vi "诊断标定3 - 副本.vi"(8 "CAN端口":u16(ring), 9 "设备索引号":u16(ring), 10 "CAN卡类型":u32(ring)=21) -> ()   [LabVIEW 2013] (continued)
              tunnel: w2286 -> [w2289 w2294]
              tunnel: [w2289 w2293] -> w2285
              frame False {
              }
              frame True {
                n1897 = local write "布尔"(TRUE ("布尔")) -> ()
                n1898 = Enqueue Element(queue=w2296, element="读配置文件", error in (no error)=w2294) -> (queue out=w2295:refnum<queue>, error out=w2293:errorcluster)  [unwired: 2 out]
                n1899 = call <vilib>:"Set Busy.vi"() -> ()  [unwired: 4 in, 8 out]
              }
            }
          }
          event "保存主板参数": Value Change {
            n1900 = event-data() -> ("NewVal"=w2297:bool)  [unwired: 6 out]
            n1901 = case shown="真" w2297 {
              tunnel: w2301 -> [w2303 w2308]
              tunnel: [w2303 w2307] -> w2300
              tunnel: w2299 -> [w2302 w2306]
              tunnel: [w2302 w2305] -> w2298
              frame False {
              }
              frame True {
                n1902 = call <vilib>:"Set Busy.vi"() -> ()  [unwired: 4 in, 8 out]
                n1903 = Enqueue Element(queue=w2308, element="写配置文件", error in (no error)=w2306) -> (queue out=w2307:refnum<queue>, error out=w2305:errorcluster)  [unwired: 2 out]
              }
            }
          }
          event "继电器全开": Value Change {
            n1904 = event-data() -> ("NewVal"=w2309:bool)  [unwired: 6 out]
            n1905 = case shown="真" w2309 {
              tunnel: w2309 -> [_ w2312]
              frame False {
              }
              frame True {
                n1906 = stacked-sequence {
                  tunnel: w2312 -> [_ w2322 _]
                  frame #0 {
                    w2313 = FALSE ("清BUFF")
                    n1907 = local write "正级继电器"(w2313) -> ()
                    n1908 = local write "负级继电器"(w2313) -> ()
                    n1909 = local write "充电继电器"(w2313) -> ()
                    n1910 = local write "加热继电器"(w2313) -> ()
                    n1911 = local write "风机继电器"(w2313) -> ()
                    n1912 = local write "预充电继电器"(w2313) -> ()
                    n1913 = local write "继电器超时处理"(FALSE ("继电器超时处理")) -> ()
                    n1914 = local write "主从选择"(enum32{"主板", "从板"}."主板" ("主从选择")) -> ()
                    n1915 = local write "清BUFF"(FALSE ("清BUFF")) -> ()
                  }
                  frame #1 {
                    n1916 = case shown="真" w2322 {
                      selector: w2322 -> [_ w2337]
                      frame False {
                      }
                      frame True {
                        w2333 = 256.0 ("y")
                        w2324 = u32 1 ("命令序号")
                        w2323 = u8 192 ("命令")
                        n1917 = local read "动作保持时间"() -> (w2334:dbl)
                        n1918 = Quotient & Remainder(x=w2334, y=w2333) -> (x-y*floor(x/y)=w2326:dbl, floor(x/y)=w2330:dbl)
                        n1919 = Quotient & Remainder(x=w2330, y=w2333) -> (x-y*floor(x/y)=w2327:dbl, floor(x/y)=w2331:dbl)
                        n1920 = Quotient & Remainder(x=w2331, y=w2333) -> (x-y*floor(x/y)=w2328:dbl, floor(x/y)=w2332:dbl)
                        n1921 = local read "设备索引号"() -> (w2341:u16)
                        n1922 = local read "CAN卡类型"() -> (w2342:u32)
                        n1923 = local read "CAN端口"() -> (w2340:u16)
                        n1924 = Boolean To (0,1)(Boolean=w2337) -> (0, 1=w2335:i16)
                        n1925 = Quotient & Remainder(x=w2332, y=w2333) -> (x-y*floor(x/y)=w2329:dbl)  [unwired: 1 out]
                        n1926 = Build Array(i16 170 ("元素"), w2335, w2329, w2328, w2327, w2326, 0.0 ("元素")) -> (w2338:dbl[])
                        n1927 = call "多帧发送机制(EV05).vi"("can卡类型"=w2342, "设备索引号"=w2341, "CAN端口"=w2340, "命令"=w2323, "板号"=u8 0, "命令序号"=w2324, "输入数据"=w2338) -> ()  [unwired: 1 in, 12 out]
                        n1928 = local write "命令序号"(w2324) -> ()
                        n1929 = local write "命令"(w2323) -> ()
                      }
                    }
                    n1930 = local write "控制1"(TRUE ("控制1")) -> ()
                    n1931 = local write "写?"(FALSE ("写?")) -> ()
                    n1932 = local write "消除"(TRUE ("消除")) -> ()
                    n1933 = global write "EV05全局变量1.vi" "流控帧 2"(TRUE ("流控帧 2")) -> ()
                    n1934 = global write "EV05全局变量1.vi" "流控帧"(FALSE ("流控帧")) -> ()
                  }
                  frame #2 {
                    n1935 = flat-sequence {
                      tunnel: [w2344] -> w2343
                      tunnel: w2343 -> [w2351]
                      frame #0 {
                        n1936 = while {
                          tunnel: [w2345] -> w2344
                          i -> [w2349]
                          stop <- w2346 stop-if-true
                          n1937 = local read "继电器超时处理"() -> (w2345:bool)
                          n1938 = Greater Or Equal?(x=w2349, y=20) -> (x >= y?=w2347:bool)
                          n1939 = Wait Until Next ms Multiple(millisecond multiple=u32 100 ("毫秒倍数")) -> ()  [unwired: 1 out]
                          n1940 = Or(x=w2345, y=w2347) -> (x .or. y?=w2346:bool)
                        }
                      }
                      frame #1 {
                        n1941 = case shown="真" w2351 {
                          frame False {
                            n1942 = One Button Dialog(message="继电器处理超时" ("消息"), button name ("OK")="是" ("按钮名称（“确定”）")) -> ()  [unwired: 1 out]
                          }
                          frame True {
                            w2354 = TRUE ("清BUFF")
                            n1943 = local write "正级继电器"(w2354) -> ()
                            n1944 = local write "负级继电器"(w2354) -> ()
                            n1945 = local write "充电继电器"(w2354) -> ()
                            n1946 = local write "加热继电器"(w2354) -> ()
                            n1947 = local write "风机继电器"(w2354) -> ()
                            n1948 = local write "预充电继电器"(w2354) -> ()
                          }
                        }
                      }
                    }
                  }
                }
              }
            }
          }
          event "继电器全关": Value Change {
            n1949 = event-data() -> ("NewVal"=w2355:bool)  [unwired: 6 out]
            n1950 = case shown="真" w2355 {
              tunnel: w2355 -> [_ w2358]
              frame False {
              }
              frame True {
                n1951 = stacked-sequence {
                  tunnel: w2358 -> [_ w2368 _]
                  frame #0 {
                    w2359 = TRUE ("清BUFF")
                    n1952 = local write "正级继电器"(w2359) -> ()
                    n1953 = local write "负级继电器"(w2359) -> ()
                    n1954 = local write "充电继电器"(w2359) -> ()
                    n1955 = local write "加热继电器"(w2359) -> ()
                    n1956 = local write "风机继电器"(w2359) -> ()
                    n1957 = local write "预充电继电器"(w2359) -> ()
                    n1958 = local write "继电器超时处理"(FALSE ("继电器超时处理")) -> ()
                    n1959 = local write "主从选择"(enum32{"主板", "从板"}."主板" ("主从选择")) -> ()
                    n1960 = global write "EV05全局变量1.vi" "流控帧"(FALSE ("流控帧")) -> ()
                    n1961 = local write "清BUFF"(FALSE ("清BUFF")) -> ()
                  }
                  frame #1 {
                    n1962 = case shown="真" w2368 {
                      selector: w2368 -> [_ w2383]
                      frame False {
                      }
                      frame True {
                        w2379 = 256.0 ("y")
                        w2370 = u32 1 ("命令序号")
                        w2369 = u8 192 ("命令")
                        n1963 = local read "动作保持时间"() -> (w2380:dbl)
                        n1964 = Quotient & Remainder(x=w2380, y=w2379) -> (x-y*floor(x/y)=w2372:dbl, floor(x/y)=w2376:dbl)
                        n1965 = Quotient & Remainder(x=w2376, y=w2379) -> (x-y*floor(x/y)=w2373:dbl, floor(x/y)=w2377:dbl)
                        n1966 = Quotient & Remainder(x=w2377, y=w2379) -> (x-y*floor(x/y)=w2374:dbl, floor(x/y)=w2378:dbl)
                        n1967 = local read "设备索引号"() -> (w2387:u16)
                        n1968 = local read "CAN卡类型"() -> (w2388:u32)
                        n1969 = local read "CAN端口"() -> (w2386:u16)
                        n1970 = Boolean To (0,1)(Boolean=w2383) -> (0, 1=w2381:i16)
                        n1971 = Quotient & Remainder(x=w2378, y=w2379) -> (x-y*floor(x/y)=w2375:dbl)  [unwired: 1 out]
                        n1972 = Build Array(i16 85 ("元素"), w2381, w2375, w2374, w2373, w2372, 0.0 ("元素")) -> (w2384:dbl[])
                        n1973 = call "多帧发送机制(EV05).vi"("can卡类型"=w2388, "设备索引号"=w2387, "CAN端口"=w2386, "命令"=w2369, "板号"=u8 0, "命令序号"=w2370, "输入数据"=w2384) -> ()  [unwired: 1 in, 12 out]
                        n1974 = local write "命令序号"(w2370) -> ()
                        n1975 = local write "命令"(w2369) -> ()
                      }
                    }
                    n1976 = local write "控制1"(TRUE ("控制1")) -> ()
                    n1977 = local write "写?"(FALSE ("写?")) -> ()
                    n1978 = local write "消除"(TRUE ("消除")) -> ()
                    n1979 = global write "EV05全局变量1.vi" "流控帧 2"(TRUE ("流控帧 2")) -> ()
                  }
                  frame #2 {
                    n1980 = flat-sequence {
                      tunnel: [w2390] -> w2389
                      tunnel: w2389 -> [w2397]
                      frame #0 {
                        n1981 = while {
                          tunnel: [w2391] -> w2390
                          i -> [w2395]
                          stop <- w2392 stop-if-true
                          n1982 = local read "继电器超时处理"() -> (w2391:bool)
                          n1983 = Greater Or Equal?(x=w2395, y=20) -> (x >= y?=w2393:bool)
                          n1984 = Wait Until Next ms Multiple(millisecond multiple=u32 100 ("毫秒倍数")) -> ()  [unwired: 1 out]
                          n1985 = Or(x=w2391, y=w2393) -> (x .or. y?=w2392:bool)
                        }
                      }
                      frame #1 {
                        n1986 = case shown="真" w2397 {
                          frame False {
                            n1987 = One Button Dialog(message="继电器处理超时" ("消息"), button name ("OK")="是" ("按钮名称（“确定”）")) -> ()  [unwired: 1 out]
                          }
                          frame True {
                            w2400 = FALSE ("清BUFF")
                            n1988 = local write "正级继电器"(w2400) -> ()
                            n1989 = local write "负级继电器"(w2400) -> ()
                            n1990 = local write "充电继电器"(w2400) -> ()
                            n1991 = local write "加热继电器"(w2400) -> ()
                            n1992 = local write "风机继电器"(w2400) -> ()
                            n1993 = local write "预充电继电器"(w2400) -> ()
                          }
                        }
                      }
                    }
                  }
                }
              }
            }
          }
          event "控制按键全为开": Value Change {
            n1994 = event-data() -> ("NewVal"=w2401:bool)  [unwired: 6 out]
            n1995 = case shown="真" w2401 {
              frame False {
              }
              frame True {
                w2402 = TRUE ("正级继电器")
                n1996 = local write "加热继电器(从)"(w2402) -> ()
                n1997 = local write "风机继电器(从)"(w2402) -> ()
                n1998 = local write "DO1 2"(w2402) -> ()
                n1999 = local write "DO1"(w2402) -> ()
                n2000 = local write "DO2"(w2402) -> ()
                n2001 = local write "正级继电器"(w2402) -> ()
                n2002 = local write "负级继电器"(w2402) -> ()
                n2003 = local write "加热继电器"(w2402) -> ()
                n2004 = local write "预充电继电器"(w2402) -> ()
                n2005 = local write "充电继电器"(w2402) -> ()
                n2006 = local write "风机继电器"(w2402) -> ()
              }
            }
          }
          event "控制按键全为关": Value Change {
            n2007 = event-data() -> ("NewVal"=w2403:bool)  [unwired: 6 out]
            n2008 = case shown="真" w2403 {
              frame False {
              }
              frame True {
                w2404 = FALSE ("正级继电器")
                n2009 = local write "加热继电器(从)"(w2404) -> ()
                n2010 = local write "风机继电器(从)"(w2404) -> ()
                n2011 = local write "DO1 2"(w2404) -> ()
                n2012 = local write "DO1"(w2404) -> ()
                n2013 = local write "DO2"(w2404) -> ()
                n2014 = local write "正级继电器"(w2404) -> ()
                n2015 = local write "负级继电器"(w2404) -> ()
                n2016 = local write "加热继电器"(w2404) -> ()
                n2017 = local write "预充电继电器"(w2404) -> ()
                n2018 = local write "充电继电器"(w2404) -> ()
                n2019 = local write "风机继电器"(w2404) -> ()
              }
            }
          }
          event "正级继电器": Value Change {
            n2020 = event-data() -> ("NewVal"=w2405:bool)  [unwired: 6 out]
            n2021 = stacked-sequence {
              tunnel: w2405 -> [_ w2418 _]
              frame #0 {
                w2408 = FALSE ("清BUFF")
                n2022 = local write "继电器超时处理"(FALSE ("继电器超时处理")) -> ()
                n2023 = local write "主从选择"(enum32{"主板", "从板"}."主板" ("主从选择")) -> ()
                n2024 = local write "正级继电器 12"(w2408) -> ()
                n2025 = local write "清BUFF"(w2408) -> ()
              }
              frame #1 {
                n2026 = case shown="假" w2418 {
                  selector: w2418 -> [w2433 w2453]
                  tunnel: [w2432 w2452] -> w2417
                  tunnel: [w2420 w2440] -> w2412
                  frame False {
                    w2428 = 256.0 ("y")
                    w2420 = u32 1 ("命令序号")
                    w2432 = u8 192 ("命令")
                    n2027 = local read "动作保持时间"() -> (w2429:dbl)
                    n2028 = Quotient & Remainder(x=w2429, y=w2428) -> (x-y*floor(x/y)=w2421:dbl, floor(x/y)=w2425:dbl)
                    n2029 = Quotient & Remainder(x=w2425, y=w2428) -> (x-y*floor(x/y)=w2422:dbl, floor(x/y)=w2426:dbl)
                    n2030 = Quotient & Remainder(x=w2426, y=w2428) -> (x-y*floor(x/y)=w2423:dbl, floor(x/y)=w2427:dbl)
                    n2031 = local read "设备索引号"() -> (w2437:u16)
                    n2032 = local read "CAN卡类型"() -> (w2438:u32)
                    n2033 = local read "CAN端口"() -> (w2436:u16)
                    n2034 = Boolean To (0,1)(Boolean=w2433) -> (0, 1=w2430:i16)
                    n2035 = Quotient & Remainder(x=w2427, y=w2428) -> (x-y*floor(x/y)=w2424:dbl)  [unwired: 1 out]
                    n2036 = Build Array(i16 1 ("元素"), w2430, w2424, w2423, w2422, w2421, 0.0 ("元素")) -> (w2434:dbl[])
                    n2037 = call "多帧发送机制(EV05).vi"("can卡类型"=w2438, "设备索引号"=w2437, "CAN端口"=w2436, "命令"=w2432, "板号"=u8 0, "命令序号"=w2420, "输入数据"=w2434) -> ()  [unwired: 1 in, 12 out]
                  }
                  frame True {
                    w2448 = 256.0 ("y")
                    w2440 = u32 1 ("命令序号")
                    w2452 = u8 192 ("命令")
                    n2038 = local read "动作保持时间"() -> (w2449:dbl)
                    n2039 = Quotient & Remainder(x=w2449, y=w2448) -> (x-y*floor(x/y)=w2441:dbl, floor(x/y)=w2445:dbl)
                    n2040 = Quotient & Remainder(x=w2445, y=w2448) -> (x-y*floor(x/y)=w2442:dbl, floor(x/y)=w2446:dbl)
                    n2041 = Quotient & Remainder(x=w2446, y=w2448) -> (x-y*floor(x/y)=w2443:dbl, floor(x/y)=w2447:dbl)
                    n2042 = local read "设备索引号"() -> (w2457:u16)
                    n2043 = local read "CAN卡类型"() -> (w2458:u32)
                    n2044 = local read "CAN端口"() -> (w2456:u16)
                    n2045 = Boolean To (0,1)(Boolean=w2453) -> (0, 1=w2450:i16)
                    n2046 = Quotient & Remainder(x=w2447, y=w2448) -> (x-y*floor(x/y)=w2444:dbl)  [unwired: 1 out]
                    n2047 = Build Array(i16 1 ("元素"), w2450, w2444, w2443, w2442, w2441, 0.0 ("元素")) -> (w2454:dbl[])
                    n2048 = call "多帧发送机制(EV05).vi"("can卡类型"=w2458, "设备索引号"=w2457, "CAN端口"=w2456, "命令"=w2452, "板号"=u8 0, "命令序号"=w2440, "输入数据"=w2454) -> ()  [unwired: 1 in, 12 out]
                  }
                }
                n2049 = local write "命令序号"(w2412) -> ()
                n2050 = local write "命令"(w2417) -> ()
                n2051 = local write "控制1"(TRUE ("控制1")) -> ()
                n2052 = local write "写?"(FALSE ("写?")) -> ()
                n2053 = global write "EV05全局变量1.vi" "流控帧"(FALSE ("流控帧")) -> ()
                n2054 = local write "消除"(TRUE ("消除")) -> ()
                n2055 = global write "EV05全局变量1.vi" "流控帧 2"(TRUE ("流控帧 2")) -> ()
              }
              frame #2 {
                n2056 = flat-sequence {
                  tunnel: [w2460] -> w2459
                  tunnel: w2459 -> [w2467]
                  frame #0 {
                    n2057 = while {
                      tunnel: [w2461] -> w2460
                      i -> [w2465]
                      stop <- w2462 stop-if-true
                      n2058 = local read "继电器超时处理"() -> (w2461:bool)
                      n2059 = Greater Or Equal?(x=w2465, y=20) -> (x >= y?=w2463:bool)
                      n2060 = Wait Until Next ms Multiple(millisecond multiple=u32 100 ("毫秒倍数")) -> ()  [unwired: 1 out]
                      n2061 = Or(x=w2461, y=w2463) -> (x .or. y?=w2462:bool)
                    }
                  }
                  frame #1 {
                    n2062 = case shown="假" w2467 {
                      frame False {
                        n2063 = local read "正级继电器"() -> (w2469:bool)
                        n2064 = Not(x=w2469) -> (.not. x?=w2468:bool)
                        n2065 = local write "正级继电器"(w2468) -> ()
                        n2066 = One Button Dialog(message="继电器处理超时" ("消息"), button name ("OK")="是" ("按钮名称（“确定”）")) -> ()  [unwired: 1 out]
                      }
                      frame True {
                      }
                    }
                  }
                }
              }
            }
          }
          event "负级继电器": Value Change {
            n2067 = event-data() -> ("NewVal"=w2472:bool)  [unwired: 6 out]
            n2068 = stacked-sequence {
              tunnel: w2472 -> [_ w2485 _]
              frame #0 {
                w2475 = FALSE ("继电器超时处理")
                n2069 = local write "继电器超时处理"(w2475) -> ()
                n2070 = local write "正级继电器 2"(w2475) -> ()
                n2071 = local write "主从选择"(enum32{"主板", "从板"}."主板" ("主从选择")) -> ()
              }
              frame #1 {
                n2072 = case shown="假" w2485 {
                  selector: w2485 -> [w2499 w2519]
                  tunnel: [w2498 w2518] -> w2484
                  tunnel: [w2487 w2507] -> w2479
                  frame False {
                    w2495 = 256.0 ("y")
                    w2487 = u32 1 ("命令序号")
                    w2498 = u8 192 ("命令")
                    n2073 = local read "动作保持时间"() -> (w2496:dbl)
                    n2074 = Quotient & Remainder(x=w2496, y=w2495) -> (x-y*floor(x/y)=w2488:dbl, floor(x/y)=w2492:dbl)
                    n2075 = Quotient & Remainder(x=w2492, y=w2495) -> (x-y*floor(x/y)=w2489:dbl, floor(x/y)=w2493:dbl)
                    n2076 = Quotient & Remainder(x=w2493, y=w2495) -> (x-y*floor(x/y)=w2490:dbl, floor(x/y)=w2494:dbl)
                    n2077 = Quotient & Remainder(x=w2494, y=w2495) -> (x-y*floor(x/y)=w2491:dbl)  [unwired: 1 out]
                    n2078 = Boolean To (0,1)(Boolean=w2499) -> (0, 1=w2497:i16)
                    n2079 = local read "设备索引号"() -> (w2504:u16)
                    n2080 = local read "CAN卡类型"() -> (w2505:u32)
                    n2081 = local read "CAN端口"() -> (w2503:u16)
                    n2082 = Build Array(i16 2 ("元素"), w2497, w2491, w2490, w2489, w2488, 0.0 ("元素")) -> (w2501:dbl[])
                    n2083 = call "多帧发送机制(EV05).vi"("can卡类型"=w2505, "设备索引号"=w2504, "CAN端口"=w2503, "命令"=w2498, "板号"=u8 0, "命令序号"=w2487, "输入数据"=w2501) -> ()  [unwired: 1 in, 12 out]
                  }
                  frame True {
                    w2515 = 256.0 ("y")
                    w2507 = u32 1 ("命令序号")
                    w2518 = u8 192 ("命令")
                    n2084 = local read "动作保持时间"() -> (w2516:dbl)
                    n2085 = Quotient & Remainder(x=w2516, y=w2515) -> (x-y*floor(x/y)=w2508:dbl, floor(x/y)=w2512:dbl)
                    n2086 = Quotient & Remainder(x=w2512, y=w2515) -> (x-y*floor(x/y)=w2509:dbl, floor(x/y)=w2513:dbl)
                    n2087 = Quotient & Remainder(x=w2513, y=w2515) -> (x-y*floor(x/y)=w2510:dbl, floor(x/y)=w2514:dbl)
                    n2088 = Quotient & Remainder(x=w2514, y=w2515) -> (x-y*floor(x/y)=w2511:dbl)  [unwired: 1 out]
                    n2089 = Boolean To (0,1)(Boolean=w2519) -> (0, 1=w2517:i16)
                    n2090 = local read "设备索引号"() -> (w2524:u16)
                    n2091 = local read "CAN卡类型"() -> (w2525:u32)
                    n2092 = local read "CAN端口"() -> (w2523:u16)
                    n2093 = Build Array(i16 2 ("元素"), w2517, w2511, w2510, w2509, w2508, 0.0 ("元素")) -> (w2521:dbl[])
                    n2094 = call "多帧发送机制(EV05).vi"("can卡类型"=w2525, "设备索引号"=w2524, "CAN端口"=w2523, "命令"=w2518, "板号"=u8 0, "命令序号"=w2507, "输入数据"=w2521) -> ()  [unwired: 1 in, 12 out]
                  }
                }
                n2095 = local write "命令"(w2484) -> ()
                n2096 = local write "命令序号"(w2479) -> ()
                n2097 = local write "清BUFF"(FALSE ("清BUFF")) -> ()
                n2098 = global write "EV05全局变量1.vi" "流控帧"(FALSE ("流控帧")) -> ()
                n2099 = local write "控制1"(TRUE ("控制1")) -> ()
                n2100 = global write "EV05全局变量1.vi" "流控帧 2"(TRUE ("流控帧 2")) -> ()
                n2101 = local write "写?"(FALSE ("写?")) -> ()
                n2102 = local write "消除"(TRUE ("消除")) -> ()
              }
              frame #2 {
                n2103 = flat-sequence {
                  tunnel: [w2527] -> w2526
                  tunnel: w2526 -> [w2534]
                  frame #0 {
                    n2104 = while {
                      tunnel: [w2528] -> w2527
                      i -> [w2532]
                      stop <- w2529 stop-if-true
                      n2105 = local read "继电器超时处理"() -> (w2528:bool)
                      n2106 = Greater Or Equal?(x=w2532, y=20) -> (x >= y?=w2530:bool)
                      n2107 = Wait Until Next ms Multiple(millisecond multiple=u32 100 ("毫秒倍数")) -> ()  [unwired: 1 out]
                      n2108 = Or(x=w2528, y=w2530) -> (x .or. y?=w2529:bool)
                    }
                  }
                  frame #1 {
                    n2109 = case shown="假" w2534 {
                      frame False {
                        n2110 = local read "负级继电器"() -> (w2535:bool)
                        n2111 = Not(x=w2535) -> (.not. x?=w2536:bool)
                        n2112 = local write "负级继电器"(w2536) -> ()
                        n2113 = One Button Dialog(message="继电器处理超时" ("消息"), button name ("OK")="是" ("按钮名称（“确定”）")) -> ()  [unwired: 1 out]
                      }
                      frame True {
                      }
                    }
                  }
                }
              }
            }
          }
          event "预充电继电器": Value Change {
            n2114 = event-data() -> ("NewVal"=w2539:bool)  [unwired: 6 out]
            n2115 = stacked-sequence {
              tunnel: w2539 -> [_ w2552 _]
              frame #0 {
                w2543 = FALSE ("继电器超时处理")
                n2116 = local write "继电器超时处理"(w2543) -> ()
                n2117 = local write "正级继电器 3"(w2543) -> ()
                n2118 = global write "EV05全局变量1.vi" "流控帧"(FALSE ("流控帧")) -> ()
                n2119 = local write "主从选择"(enum32{"主板", "从板"}."主板" ("主从选择")) -> ()
              }
              frame #1 {
                n2120 = case shown="假" w2552 {
                  selector: w2552 -> [w2566 w2586]
                  tunnel: [w2565 w2585] -> w2551
                  tunnel: [w2554 w2574] -> w2546
                  frame False {
                    w2562 = 256.0 ("y")
                    w2554 = u32 1 ("命令序号")
                    w2565 = u8 192 ("命令")
                    n2121 = local read "动作保持时间"() -> (w2563:dbl)
                    n2122 = Quotient & Remainder(x=w2563, y=w2562) -> (x-y*floor(x/y)=w2555:dbl, floor(x/y)=w2559:dbl)
                    n2123 = Quotient & Remainder(x=w2559, y=w2562) -> (x-y*floor(x/y)=w2556:dbl, floor(x/y)=w2560:dbl)
                    n2124 = Quotient & Remainder(x=w2560, y=w2562) -> (x-y*floor(x/y)=w2557:dbl, floor(x/y)=w2561:dbl)
                    n2125 = Quotient & Remainder(x=w2561, y=w2562) -> (x-y*floor(x/y)=w2558:dbl)  [unwired: 1 out]
                    n2126 = Boolean To (0,1)(Boolean=w2566) -> (0, 1=w2564:i16)
                    n2127 = local read "设备索引号"() -> (w2571:u16)
                    n2128 = local read "CAN卡类型"() -> (w2572:u32)
                    n2129 = local read "CAN端口"() -> (w2570:u16)
                    n2130 = Build Array(i16 3 ("元素"), w2564, w2558, w2557, w2556, w2555, 0.0 ("元素")) -> (w2568:dbl[])
                    n2131 = call "多帧发送机制(EV05).vi"("can卡类型"=w2572, "设备索引号"=w2571, "CAN端口"=w2570, "命令"=w2565, "板号"=u8 0, "命令序号"=w2554, "输入数据"=w2568) -> ()  [unwired: 1 in, 12 out]
                  }
                  frame True {
                    w2582 = 256.0 ("y")
                    w2574 = u32 1 ("命令序号")
                    w2585 = u8 192 ("命令")
                    n2132 = local read "动作保持时间"() -> (w2583:dbl)
                    n2133 = Quotient & Remainder(x=w2583, y=w2582) -> (x-y*floor(x/y)=w2575:dbl, floor(x/y)=w2579:dbl)
                    n2134 = Quotient & Remainder(x=w2579, y=w2582) -> (x-y*floor(x/y)=w2576:dbl, floor(x/y)=w2580:dbl)
                    n2135 = Quotient & Remainder(x=w2580, y=w2582) -> (x-y*floor(x/y)=w2577:dbl, floor(x/y)=w2581:dbl)
                    n2136 = Quotient & Remainder(x=w2581, y=w2582) -> (x-y*floor(x/y)=w2578:dbl)  [unwired: 1 out]
                    n2137 = Boolean To (0,1)(Boolean=w2586) -> (0, 1=w2584:i16)
                    n2138 = local read "设备索引号"() -> (w2591:u16)
                    n2139 = local read "CAN卡类型"() -> (w2592:u32)
                    n2140 = local read "CAN端口"() -> (w2590:u16)
                    n2141 = Build Array(i16 3 ("元素"), w2584, w2578, w2577, w2576, w2575, 0.0 ("元素")) -> (w2588:dbl[])
                    n2142 = call "多帧发送机制(EV05).vi"("can卡类型"=w2592, "设备索引号"=w2591, "CAN端口"=w2590, "命令"=w2585, "板号"=u8 0, "命令序号"=w2574, "输入数据"=w2588) -> ()  [unwired: 1 in, 12 out]
                  }
                }
                n2143 = local write "命令序号"(w2546) -> ()
                n2144 = local write "清BUFF"(FALSE ("清BUFF")) -> ()
                n2145 = local write "控制1"(TRUE ("控制1")) -> ()
                n2146 = global write "EV05全局变量1.vi" "流控帧 2"(TRUE ("流控帧 2")) -> ()
                n2147 = local write "消除"(TRUE ("消除")) -> ()
                n2148 = local write "命令"(w2551) -> ()
                n2149 = local write "写?"(FALSE ("写?")) -> ()
              }
              frame #2 {
                n2150 = flat-sequence {
                  tunnel: [w2594] -> w2593
                  tunnel: w2593 -> [w2601]
                  frame #0 {
                    n2151 = while {
                      tunnel: [w2595] -> w2594
                      i -> [w2599]
                      stop <- w2596 stop-if-true
                      n2152 = local read "继电器超时处理"() -> (w2595:bool)
                      n2153 = Greater Or Equal?(x=w2599, y=20) -> (x >= y?=w2597:bool)
                      n2154 = Wait Until Next ms Multiple(millisecond multiple=u32 100 ("毫秒倍数")) -> ()  [unwired: 1 out]
                      n2155 = Or(x=w2595, y=w2597) -> (x .or. y?=w2596:bool)
                    }
                  }
                  frame #1 {
                    n2156 = case shown="假" w2601 {
                      frame False {
                        n2157 = local read "预充电继电器"() -> (w2602:bool)
                        n2158 = Not(x=w2602) -> (.not. x?=w2603:bool)
                        n2159 = local write "预充电继电器"(w2603) -> ()
                        n2160 = One Button Dialog(message="继电器处理超时" ("消息"), button name ("OK")="是" ("按钮名称（“确定”）")) -> ()  [unwired: 1 out]
                      }
                      frame True {
                      }
                    }
                  }
                }
              }
            }
          }
          event "加热继电器": Value Change {
            n2161 = event-data() -> ("NewVal"=w2606:bool)  [unwired: 6 out]
            n2162 = stacked-sequence {
              tunnel: w2606 -> [_ w2619 _]
              frame #0 {
                w2610 = FALSE ("继电器超时处理")
                n2163 = local write "继电器超时处理"(w2610) -> ()
                n2164 = local write "正级继电器 5"(w2610) -> ()
                n2165 = global write "EV05全局变量1.vi" "流控帧"(FALSE ("流控帧")) -> ()
                n2166 = local write "主从选择"(enum32{"主板", "从板"}."主板" ("主从选择")) -> ()
              }
              frame #1 {
                n2167 = case shown="假" w2619 {
                  selector: w2619 -> [w2633 w2653]
                  tunnel: [w2632 w2652] -> w2618
                  tunnel: [w2621 w2641] -> w2613
                  frame False {
                    w2629 = 256.0 ("y")
                    w2621 = u32 1 ("命令序号")
                    w2632 = u8 192 ("命令")
                    n2168 = local read "动作保持时间"() -> (w2630:dbl)
                    n2169 = Quotient & Remainder(x=w2630, y=w2629) -> (x-y*floor(x/y)=w2622:dbl, floor(x/y)=w2626:dbl)
                    n2170 = Quotient & Remainder(x=w2626, y=w2629) -> (x-y*floor(x/y)=w2623:dbl, floor(x/y)=w2627:dbl)
                    n2171 = Quotient & Remainder(x=w2627, y=w2629) -> (x-y*floor(x/y)=w2624:dbl, floor(x/y)=w2628:dbl)
                    n2172 = Quotient & Remainder(x=w2628, y=w2629) -> (x-y*floor(x/y)=w2625:dbl)  [unwired: 1 out]
                    n2173 = Boolean To (0,1)(Boolean=w2633) -> (0, 1=w2631:i16)
                    n2174 = local read "设备索引号"() -> (w2638:u16)
                    n2175 = local read "CAN卡类型"() -> (w2639:u32)
                    n2176 = local read "CAN端口"() -> (w2637:u16)
                    n2177 = Build Array(i16 4 ("元素"), w2631, w2625, w2624, w2623, w2622, 0.0 ("元素")) -> (w2635:dbl[])
                    n2178 = call "多帧发送机制(EV05).vi"("can卡类型"=w2639, "设备索引号"=w2638, "CAN端口"=w2637, "命令"=w2632, "板号"=u8 0, "命令序号"=w2621, "输入数据"=w2635) -> ()  [unwired: 1 in, 12 out]
                  }
                  frame True {
                    w2649 = 256.0 ("y")
                    w2641 = u32 1 ("命令序号")
                    w2652 = u8 192 ("命令")
                    n2179 = local read "动作保持时间"() -> (w2650:dbl)
                    n2180 = Quotient & Remainder(x=w2650, y=w2649) -> (x-y*floor(x/y)=w2642:dbl, floor(x/y)=w2646:dbl)
                    n2181 = Quotient & Remainder(x=w2646, y=w2649) -> (x-y*floor(x/y)=w2643:dbl, floor(x/y)=w2647:dbl)
                    n2182 = Quotient & Remainder(x=w2647, y=w2649) -> (x-y*floor(x/y)=w2644:dbl, floor(x/y)=w2648:dbl)
                    n2183 = Quotient & Remainder(x=w2648, y=w2649) -> (x-y*floor(x/y)=w2645:dbl)  [unwired: 1 out]
                    n2184 = Boolean To (0,1)(Boolean=w2653) -> (0, 1=w2651:i16)
                    n2185 = local read "设备索引号"() -> (w2658:u16)
                    n2186 = local read "CAN卡类型"() -> (w2659:u32)
                    n2187 = local read "CAN端口"() -> (w2657:u16)
                    n2188 = Build Array(i16 4 ("元素"), w2651, w2645, w2644, w2643, w2642, 0.0 ("元素")) -> (w2655:dbl[])
                    n2189 = call "多帧发送机制(EV05).vi"("can卡类型"=w2659, "设备索引号"=w2658, "CAN端口"=w2657, "命令"=w2652, "板号"=u8 0, "命令序号"=w2641, "输入数据"=w2655) -> ()  [unwired: 1 in, 12 out]
                  }
                }
                n2190 = local write "命令序号"(w2613) -> ()
                n2191 = local write "清BUFF"(FALSE ("清BUFF")) -> ()
                n2192 = local write "命令"(w2618) -> ()
                n2193 = local write "控制1"(TRUE ("控制1")) -> ()
                n2194 = local write "写?"(FALSE ("写?")) -> ()
                n2195 = global write "EV05全局变量1.vi" "流控帧 2"(TRUE ("流控帧 2")) -> ()
                n2196 = local write "消除"(TRUE ("消除")) -> ()
              }
              frame #2 {
                n2197 = flat-sequence {
                  tunnel: [w2661] -> w2660
                  tunnel: w2660 -> [w2668]
                  frame #0 {
                    n2198 = while {
                      tunnel: [w2662] -> w2661
                      i -> [w2666]
                      stop <- w2663 stop-if-true
                      n2199 = local read "继电器超时处理"() -> (w2662:bool)
                      n2200 = Greater Or Equal?(x=w2666, y=20) -> (x >= y?=w2664:bool)
                      n2201 = Wait Until Next ms Multiple(millisecond multiple=u32 100 ("毫秒倍数")) -> ()  [unwired: 1 out]
                      n2202 = Or(x=w2662, y=w2664) -> (x .or. y?=w2663:bool)
                    }
                  }
                  frame #1 {
                    n2203 = case shown="假" w2668 {
                      frame False {
                        n2204 = local read "加热继电器"() -> (w2669:bool)
                        n2205 = Not(x=w2669) -> (.not. x?=w2670:bool)
                        n2206 = local write "加热继电器"(w2670) -> ()
                        n2207 = One Button Dialog(message="继电器处理超时" ("消息"), button name ("OK")="是" ("按钮名称（“确定”）")) -> ()  [unwired: 1 out]
                      }
                      frame True {
                      }
                    }
                  }
                }
              }
            }
          }
          event "充电继电器": Value Change {
            n2208 = event-data() -> ("NewVal"=w2673:bool)  [unwired: 6 out]
            n2209 = stacked-sequence {
              tunnel: w2673 -> [_ w2686 _]
              frame #0 {
                w2677 = FALSE ("继电器超时处理")
                n2210 = local write "主从选择"(enum32{"主板", "从板"}."主板" ("主从选择")) -> ()
                n2211 = global write "EV05全局变量1.vi" "流控帧"(FALSE ("流控帧")) -> ()
                n2212 = local write "继电器超时处理"(w2677) -> ()
                n2213 = local write "正级继电器 4"(w2677) -> ()
              }
              frame #1 {
                n2214 = case shown="假" w2686 {
                  selector: w2686 -> [w2700 w2720]
                  tunnel: [w2699 w2719] -> w2685
                  tunnel: [w2688 w2708] -> w2680
                  frame False {
                    w2696 = 256.0 ("y")
                    w2688 = u32 1 ("命令序号")
                    w2699 = u8 192 ("命令")
                    n2215 = local read "动作保持时间"() -> (w2697:dbl)
                    n2216 = Quotient & Remainder(x=w2697, y=w2696) -> (x-y*floor(x/y)=w2689:dbl, floor(x/y)=w2693:dbl)
                    n2217 = Quotient & Remainder(x=w2693, y=w2696) -> (x-y*floor(x/y)=w2690:dbl, floor(x/y)=w2694:dbl)
                    n2218 = Quotient & Remainder(x=w2694, y=w2696) -> (x-y*floor(x/y)=w2691:dbl, floor(x/y)=w2695:dbl)
                    n2219 = Quotient & Remainder(x=w2695, y=w2696) -> (x-y*floor(x/y)=w2692:dbl)  [unwired: 1 out]
                    n2220 = Boolean To (0,1)(Boolean=w2700) -> (0, 1=w2698:i16)
                    n2221 = local read "设备索引号"() -> (w2705:u16)
                    n2222 = local read "CAN卡类型"() -> (w2706:u32)
                    n2223 = local read "CAN端口"() -> (w2704:u16)
                    n2224 = Build Array(i16 5 ("元素"), w2698, w2692, w2691, w2690, w2689, 0.0 ("元素")) -> (w2702:dbl[])
                    n2225 = call "多帧发送机制(EV05).vi"("can卡类型"=w2706, "设备索引号"=w2705, "CAN端口"=w2704, "命令"=w2699, "板号"=u8 0, "命令序号"=w2688, "输入数据"=w2702) -> ()  [unwired: 1 in, 12 out]
                  }
                  frame True {
                    w2716 = 256.0 ("y")
                    w2708 = u32 1 ("命令序号")
                    w2719 = u8 192 ("命令")
                    n2226 = local read "动作保持时间"() -> (w2717:dbl)
                    n2227 = Quotient & Remainder(x=w2717, y=w2716) -> (x-y*floor(x/y)=w2709:dbl, floor(x/y)=w2713:dbl)
                    n2228 = Quotient & Remainder(x=w2713, y=w2716) -> (x-y*floor(x/y)=w2710:dbl, floor(x/y)=w2714:dbl)
                    n2229 = Quotient & Remainder(x=w2714, y=w2716) -> (x-y*floor(x/y)=w2711:dbl, floor(x/y)=w2715:dbl)
                    n2230 = Quotient & Remainder(x=w2715, y=w2716) -> (x-y*floor(x/y)=w2712:dbl)  [unwired: 1 out]
                    n2231 = Boolean To (0,1)(Boolean=w2720) -> (0, 1=w2718:i16)
                    n2232 = local read "设备索引号"() -> (w2725:u16)
                    n2233 = local read "CAN卡类型"() -> (w2726:u32)
                    n2234 = local read "CAN端口"() -> (w2724:u16)
                    n2235 = Build Array(i16 5 ("元素"), w2718, w2712, w2711, w2710, w2709, 0.0 ("元素")) -> (w2722:dbl[])
                    n2236 = call "多帧发送机制(EV05).vi"("can卡类型"=w2726, "设备索引号"=w2725, "CAN端口"=w2724, "命令"=w2719, "板号"=u8 0, "命令序号"=w2708, "输入数据"=w2722) -> ()  [unwired: 1 in, 12 out]
                  }
                }
                n2237 = local write "命令序号"(w2680) -> ()
                n2238 = local write "命令"(w2685) -> ()
                n2239 = local write "清BUFF"(FALSE ("清BUFF")) -> ()
                n2240 = local write "控制1"(TRUE ("控制1")) -> ()
                n2241 = global write "EV05全局变量1.vi" "流控帧 2"(TRUE ("流控帧 2")) -> ()
                n2242 = local write "写?"(FALSE ("写?")) -> ()
                n2243 = local write "消除"(TRUE ("消除")) -> ()
              }
              frame #2 {
                n2244 = flat-sequence {
                  tunnel: [w2728] -> w2727
                  tunnel: w2727 -> [w2735]
                  frame #0 {
                    n2245 = while {
                      tunnel: [w2729] -> w2728
                      i -> [w2733]
                      stop <- w2730 stop-if-true
                      n2246 = local read "继电器超时处理"() -> (w2729:bool)
                      n2247 = Greater Or Equal?(x=w2733, y=20) -> (x >= y?=w2731:bool)
                      n2248 = Wait Until Next ms Multiple(millisecond multiple=u32 100 ("毫秒倍数")) -> ()  [unwired: 1 out]
                      n2249 = Or(x=w2729, y=w2731) -> (x .or. y?=w2730:bool)
                    }
                  }
                  frame #1 {
                    n2250 = case shown="假" w2735 {
                      frame False {
                        n2251 = local read "充电继电器"() -> (w2736:bool)
                        n2252 = Not(x=w2736) -> (.not. x?=w2737:bool)
                        n2253 = local write "充电继电器"(w2737) -> ()
                        n2254 = One Button Dialog(message="继电器处理超时" ("消息"), button name ("OK")="是" ("按钮名称（“确定”）")) -> ()  [unwired: 1 out]
                      }
                      frame True {
                      }
                    }
                  }
                }
              }
            }
          }
          event "风机继电器": Value Change {
            n2255 = event-data() -> ("NewVal"=w2740:bool)  [unwired: 6 out]
            n2256 = stacked-sequence {
              tunnel: w2740 -> [_ w2753 _]
              frame #0 {
                w2744 = FALSE ("继电器超时处理")
                n2257 = local write "继电器超时处理"(w2744) -> ()
                n2258 = local write "正级继电器 6"(w2744) -> ()
                n2259 = global write "EV05全局变量1.vi" "流控帧"(FALSE ("流控帧")) -> ()
                n2260 = local write "主从选择"(enum32{"主板", "从板"}."主板" ("主从选择")) -> ()
              }
              frame #1 {
                n2261 = case shown="真" w2753 {
                  selector: w2753 -> [w2767 w2787]
                  tunnel: [w2766 w2786] -> w2752
                  tunnel: [w2755 w2775] -> w2747
                  frame True {
                    w2763 = 256.0 ("y")
                    w2755 = u32 1 ("命令序号")
                    w2766 = u8 192 ("命令")
                    n2262 = local read "动作保持时间"() -> (w2764:dbl)
                    n2263 = Quotient & Remainder(x=w2764, y=w2763) -> (x-y*floor(x/y)=w2756:dbl, floor(x/y)=w2760:dbl)
                    n2264 = Quotient & Remainder(x=w2760, y=w2763) -> (x-y*floor(x/y)=w2757:dbl, floor(x/y)=w2761:dbl)
                    n2265 = Quotient & Remainder(x=w2761, y=w2763) -> (x-y*floor(x/y)=w2758:dbl, floor(x/y)=w2762:dbl)
                    n2266 = Boolean To (0,1)(Boolean=w2767) -> (0, 1=w2765:i16)
                    n2267 = local read "设备索引号"() -> (w2772:u16)
                    n2268 = local read "CAN卡类型"() -> (w2773:u32)
                    n2269 = Quotient & Remainder(x=w2762, y=w2763) -> (x-y*floor(x/y)=w2759:dbl)  [unwired: 1 out]
                    n2270 = local read "CAN端口"() -> (w2771:u16)
                    n2271 = Build Array(i16 6 ("元素"), w2765, w2759, w2758, w2757, w2756, 0.0 ("元素")) -> (w2769:dbl[])
                    n2272 = call "多帧发送机制(EV05).vi"("can卡类型"=w2773, "设备索引号"=w2772, "CAN端口"=w2771, "命令"=w2766, "板号"=u8 0, "命令序号"=w2755, "输入数据"=w2769) -> ()  [unwired: 1 in, 12 out]
                  }
                  frame False {
                    w2783 = 256.0 ("y")
                    w2775 = u32 1 ("命令序号")
                    w2786 = u8 192 ("命令")
                    n2273 = local read "动作保持时间"() -> (w2784:dbl)
                    n2274 = Quotient & Remainder(x=w2784, y=w2783) -> (x-y*floor(x/y)=w2776:dbl, floor(x/y)=w2780:dbl)
                    n2275 = Quotient & Remainder(x=w2780, y=w2783) -> (x-y*floor(x/y)=w2777:dbl, floor(x/y)=w2781:dbl)
                    n2276 = Quotient & Remainder(x=w2781, y=w2783) -> (x-y*floor(x/y)=w2778:dbl, floor(x/y)=w2782:dbl)
                    n2277 = Boolean To (0,1)(Boolean=w2787) -> (0, 1=w2785:i16)
                    n2278 = local read "设备索引号"() -> (w2792:u16)
                    n2279 = local read "CAN卡类型"() -> (w2793:u32)
                    n2280 = Quotient & Remainder(x=w2782, y=w2783) -> (x-y*floor(x/y)=w2779:dbl)  [unwired: 1 out]
                    n2281 = local read "CAN端口"() -> (w2791:u16)
                    n2282 = Build Array(i16 6 ("元素"), w2785, w2779, w2778, w2777, w2776, 0.0 ("元素")) -> (w2789:dbl[])
                    n2283 = call "多帧发送机制(EV05).vi"("can卡类型"=w2793, "设备索引号"=w2792, "CAN端口"=w2791, "命令"=w2786, "板号"=u8 0, "命令序号"=w2775, "输入数据"=w2789) -> ()  [unwired: 1 in, 12 out]
                  }
                }
                n2284 = local write "命令序号"(w2747) -> ()
                n2285 = local write "命令"(w2752) -> ()
                n2286 = local write "清BUFF"(FALSE ("清BUFF")) -> ()
                n2287 = local write "控制1"(TRUE ("控制1")) -> ()
                n2288 = global write "EV05全局变量1.vi" "流控帧 2"(TRUE ("流控帧 2")) -> ()
                n2289 = local write "写?"(FALSE ("写?")) -> ()
                n2290 = local write "消除"(TRUE ("消除")) -> ()
              }
              frame #2 {
                n2291 = flat-sequence {
                  tunnel: [w2795] -> w2794
                  tunnel: w2794 -> [w2802]
                  frame #0 {
                    n2292 = while {
                      tunnel: [w2796] -> w2795
                      i -> [w2800]
                      stop <- w2797 stop-if-true
                      n2293 = local read "继电器超时处理"() -> (w2796:bool)
                      n2294 = Greater Or Equal?(x=w2800, y=20) -> (x >= y?=w2798:bool)
                      n2295 = Wait Until Next ms Multiple(millisecond multiple=u32 100 ("毫秒倍数")) -> ()  [unwired: 1 out]
                      n2296 = Or(x=w2796, y=w2798) -> (x .or. y?=w2797:bool)
                    }
                  }
                  frame #1 {
                    n2297 = case shown="假" w2802 {
                      frame False {
                        n2298 = local read "风机继电器"() -> (w2803:bool)
                        n2299 = Not(x=w2803) -> (.not. x?=w2804:bool)
                        n2300 = local write "风机继电器"(w2804) -> ()
                        n2301 = One Button Dialog(message="继电器处理超时" ("消息"), button name ("OK")="是" ("按钮名称（“确定”）")) -> ()  [unwired: 1 out]
                      }
                      frame True {
                      }
                    }
                  }
                }
              }
            }
          }
          event "加热继电器(从)": Value Change {
            n2302 = event-data() -> ("NewVal"=w2807:bool)  [unwired: 6 out]
            n2303 = stacked-sequence {
              tunnel: w2807 -> [_ w2821 _]
              frame #0 {
                w2811 = FALSE ("继电器超时处理")
                n2304 = local write "正级继电器 7"(w2811) -> ()
                n2305 = local write "继电器超时处理"(w2811) -> ()
                n2306 = global write "EV05全局变量1.vi" "流控帧"(FALSE ("流控帧")) -> ()
                n2307 = local write "主从选择"(enum32{"主板", "从板"}."从板" ("主从选择")) -> ()
              }
              frame #1 {
                n2308 = case shown="真" w2821 {
                  selector: w2821 -> [w2836 w2856]
                  tunnel: [w2835 w2855] -> w2820
                  tunnel: [w2834 w2854] -> w2814
                  tunnel: [w2823 w2843] -> w2815
                  frame True {
                    w2831 = 256.0 ("y")
                    w2823 = u32 1 ("命令序号")
                    w2835 = u8 192 ("命令")
                    n2309 = local read "动作保持时间"() -> (w2832:dbl)
                    n2310 = Quotient & Remainder(x=w2832, y=w2831) -> (x-y*floor(x/y)=w2824:dbl, floor(x/y)=w2828:dbl)
                    n2311 = Quotient & Remainder(x=w2828, y=w2831) -> (x-y*floor(x/y)=w2825:dbl, floor(x/y)=w2829:dbl)
                    n2312 = Quotient & Remainder(x=w2829, y=w2831) -> (x-y*floor(x/y)=w2826:dbl, floor(x/y)=w2830:dbl)
                    n2313 = Quotient & Remainder(x=w2830, y=w2831) -> (x-y*floor(x/y)=w2827:dbl)  [unwired: 1 out]
                    n2314 = Boolean To (0,1)(Boolean=w2836) -> (0, 1=w2833:i16)
                    n2315 = local read "设备索引号"() -> (w2840:u16)
                    n2316 = local read "CAN卡类型"() -> (w2841:u32)
                    n2317 = local read "从板板号"() -> (w2834:u8)
                    n2318 = local read "CAN端口"() -> (w2839:u16)
                    n2319 = Build Array(i16 7 ("元素"), w2833, w2827, w2826, w2825, w2824, 0.0 ("元素")) -> (w2838:dbl[])
                    n2320 = call "多帧发送机制(EV05).vi"("can卡类型"=w2841, "设备索引号"=w2840, "CAN端口"=w2839, "命令"=w2835, "板号"=w2834, "命令序号"=w2823, "输入数据"=w2838) -> ()  [unwired: 1 in, 12 out]
                  }
                  frame False {
                    w2851 = 256.0 ("y")
                    w2843 = u32 1 ("命令序号")
                    w2855 = u8 192 ("命令")
                    n2321 = local read "动作保持时间"() -> (w2852:dbl)
                    n2322 = Quotient & Remainder(x=w2852, y=w2851) -> (x-y*floor(x/y)=w2844:dbl, floor(x/y)=w2848:dbl)
                    n2323 = Quotient & Remainder(x=w2848, y=w2851) -> (x-y*floor(x/y)=w2845:dbl, floor(x/y)=w2849:dbl)
                    n2324 = Quotient & Remainder(x=w2849, y=w2851) -> (x-y*floor(x/y)=w2846:dbl, floor(x/y)=w2850:dbl)
                    n2325 = Quotient & Remainder(x=w2850, y=w2851) -> (x-y*floor(x/y)=w2847:dbl)  [unwired: 1 out]
                    n2326 = Boolean To (0,1)(Boolean=w2856) -> (0, 1=w2853:i16)
                    n2327 = local read "设备索引号"() -> (w2860:u16)
                    n2328 = local read "CAN卡类型"() -> (w2861:u32)
                    n2329 = local read "从板板号"() -> (w2854:u8)
                    n2330 = local read "CAN端口"() -> (w2859:u16)
                    n2331 = Build Array(i16 7 ("元素"), w2853, w2847, w2846, w2845, w2844, 0.0 ("元素")) -> (w2858:dbl[])
                    n2332 = call "多帧发送机制(EV05).vi"("can卡类型"=w2861, "设备索引号"=w2860, "CAN端口"=w2859, "命令"=w2855, "板号"=w2854, "命令序号"=w2843, "输入数据"=w2858) -> ()  [unwired: 1 in, 12 out]
                  }
                }
                n2333 = local write "从板板号"(w2814) -> ()
                n2334 = local write "命令序号"(w2815) -> ()
                n2335 = local write "命令"(w2820) -> ()
                n2336 = local write "清BUFF"(FALSE ("清BUFF")) -> ()
                n2337 = local write "写?"(FALSE ("写?")) -> ()
                n2338 = local write "控制1"(TRUE ("控制1")) -> ()
                n2339 = global write "EV05全局变量1.vi" "流控帧 2"(TRUE ("流控帧 2")) -> ()
                n2340 = local write "消除"(TRUE ("消除")) -> ()
              }
              frame #2 {
                n2341 = flat-sequence {
                  tunnel: [w2863] -> w2862
                  tunnel: w2862 -> [w2870]
                  frame #0 {
                    n2342 = while {
                      tunnel: [w2864] -> w2863
                      i -> [w2868]
                      stop <- w2865 stop-if-true
                      n2343 = local read "继电器超时处理"() -> (w2864:bool)
                      n2344 = Greater Or Equal?(x=w2868, y=20) -> (x >= y?=w2866:bool)
                      n2345 = Wait Until Next ms Multiple(millisecond multiple=u32 100 ("毫秒倍数")) -> ()  [unwired: 1 out]
                      n2346 = Or(x=w2864, y=w2866) -> (x .or. y?=w2865:bool)
                    }
                  }
                  frame #1 {
                    n2347 = case shown="假" w2870 {
                      frame False {
                        n2348 = local read "加热继电器(从)"() -> (w2872:bool)
                        n2349 = Not(x=w2872) -> (.not. x?=w2871:bool)
                        n2350 = local write "加热继电器(从)"(w2871) -> ()
                        n2351 = One Button Dialog(message="继电器处理超时" ("消息"), button name ("OK")="是" ("按钮名称（“确定”）")) -> ()  [unwired: 1 out]
                      }
                      frame True {
                      }
                    }
                  }
                }
              }
            }
          }
          event "风机继电器(从)": Value Change {
            n2352 = event-data() -> ("NewVal"=w2875:bool)  [unwired: 6 out]
            n2353 = stacked-sequence {
              tunnel: w2875 -> [_ w2889 _]
              frame #0 {
                w2879 = FALSE ("继电器超时处理")
                n2354 = local write "继电器超时处理"(w2879) -> ()
                n2355 = local write "正级继电器 8"(w2879) -> ()
                n2356 = global write "EV05全局变量1.vi" "流控帧"(FALSE ("流控帧")) -> ()
                n2357 = local write "主从选择"(enum32{"主板", "从板"}."从板" ("主从选择")) -> ()
              }
              frame #1 {
                n2358 = case shown="假" w2889 {
                  selector: w2889 -> [w2904 w2924]
                  tunnel: [w2903 w2923] -> w2888
                  tunnel: [w2902 w2922] -> w2882
                  tunnel: [w2891 w2911] -> w2883
                  frame False {
                    w2899 = 256.0 ("y")
                    w2891 = u32 1 ("命令序号")
                    w2903 = u8 192 ("命令")
                    n2359 = local read "动作保持时间"() -> (w2900:dbl)
                    n2360 = Quotient & Remainder(x=w2900, y=w2899) -> (x-y*floor(x/y)=w2892:dbl, floor(x/y)=w2896:dbl)
                    n2361 = Quotient & Remainder(x=w2896, y=w2899) -> (x-y*floor(x/y)=w2893:dbl, floor(x/y)=w2897:dbl)
                    n2362 = Quotient & Remainder(x=w2897, y=w2899) -> (x-y*floor(x/y)=w2894:dbl, floor(x/y)=w2898:dbl)
                    n2363 = Quotient & Remainder(x=w2898, y=w2899) -> (x-y*floor(x/y)=w2895:dbl)  [unwired: 1 out]
                    n2364 = local read "设备索引号"() -> (w2908:u16)
                    n2365 = local read "CAN卡类型"() -> (w2909:u32)
                    n2366 = local read "从板板号"() -> (w2902:u8)
                    n2367 = Boolean To (0,1)(Boolean=w2904) -> (0, 1=w2901:i16)
                    n2368 = local read "CAN端口"() -> (w2907:u16)
                    n2369 = Build Array(i16 8 ("元素"), w2901, w2895, w2894, w2893, w2892, 0.0 ("元素")) -> (w2906:dbl[])
                    n2370 = call "多帧发送机制(EV05).vi"("can卡类型"=w2909, "设备索引号"=w2908, "CAN端口"=w2907, "命令"=w2903, "板号"=w2902, "命令序号"=w2891, "输入数据"=w2906) -> ()  [unwired: 1 in, 12 out]
                  }
                  frame True {
                    w2919 = 256.0 ("y")
                    w2911 = u32 1 ("命令序号")
                    w2923 = u8 192 ("命令")
                    n2371 = local read "动作保持时间"() -> (w2920:dbl)
                    n2372 = Quotient & Remainder(x=w2920, y=w2919) -> (x-y*floor(x/y)=w2912:dbl, floor(x/y)=w2916:dbl)
                    n2373 = Quotient & Remainder(x=w2916, y=w2919) -> (x-y*floor(x/y)=w2913:dbl, floor(x/y)=w2917:dbl)
                    n2374 = Quotient & Remainder(x=w2917, y=w2919) -> (x-y*floor(x/y)=w2914:dbl, floor(x/y)=w2918:dbl)
                    n2375 = Quotient & Remainder(x=w2918, y=w2919) -> (x-y*floor(x/y)=w2915:dbl)  [unwired: 1 out]
                    n2376 = local read "设备索引号"() -> (w2928:u16)
                    n2377 = local read "CAN卡类型"() -> (w2929:u32)
                    n2378 = local read "从板板号"() -> (w2922:u8)
                    n2379 = Boolean To (0,1)(Boolean=w2924) -> (0, 1=w2921:i16)
                    n2380 = local read "CAN端口"() -> (w2927:u16)
                    n2381 = Build Array(i16 8 ("元素"), w2921, w2915, w2914, w2913, w2912, 0.0 ("元素")) -> (w2926:dbl[])
                    n2382 = call "多帧发送机制(EV05).vi"("can卡类型"=w2929, "设备索引号"=w2928, "CAN端口"=w2927, "命令"=w2923, "板号"=w2922, "命令序号"=w2911, "输入数据"=w2926) -> ()  [unwired: 1 in, 12 out]
                  }
                }
                n2383 = local write "从板板号"(w2882) -> ()
                n2384 = local write "清BUFF"(FALSE ("清BUFF")) -> ()
                n2385 = local write "命令序号"(w2883) -> ()
                n2386 = local write "命令"(w2888) -> ()
                n2387 = local write "控制1"(TRUE ("控制1")) -> ()
                n2388 = local write "写?"(FALSE ("写?")) -> ()
                n2389 = local write "消除"(TRUE ("消除")) -> ()
                n2390 = global write "EV05全局变量1.vi" "流控帧 2"(TRUE ("流控帧 2")) -> ()
              }
              frame #2 {
                n2391 = flat-sequence {
                  tunnel: [w2931] -> w2930
                  tunnel: w2930 -> [w2938]
                  frame #0 {
                    n2392 = while {
                      tunnel: [w2932] -> w2931
                      i -> [w2936]
                      stop <- w2933 stop-if-true
                      n2393 = local read "继电器超时处理"() -> (w2932:bool)
                      n2394 = Greater Or Equal?(x=w2936, y=20) -> (x >= y?=w2934:bool)
                      n2395 = Wait Until Next ms Multiple(millisecond multiple=u32 100 ("毫秒倍数")) -> ()  [unwired: 1 out]
                      n2396 = Or(x=w2932, y=w2934) -> (x .or. y?=w2933:bool)
                    }
                  }
                  frame #1 {
                    n2397 = case shown="假" w2938 {
                      frame False {
                        n2398 = local read "风机继电器(从)"() -> (w2940:bool)
                        n2399 = Not(x=w2940) -> (.not. x?=w2939:bool)
                        n2400 = local write "风机继电器(从)"(w2939) -> ()
                        n2401 = One Button Dialog(message="继电器处理超时" ("消息"), button name ("OK")="是" ("按钮名称（“确定”）")) -> ()  [unwired: 1 out]
                      }
                      frame True {
                      }
